vi "Main.vi"() -> ()   [LabVIEW 2017]
doc: "This template is for the Queued Message Handler design pattern.\n\nThe Event Handling Loop generates messages based on user interface actions.\n\nThe Message Handling Loop processes messages generated by the Event Handling Loop, or by other messages. The messages are string values, so new messages can be added easily to the Message Cases case structure in the Message Handling Loop. Each message cluster can also provide an optional value for Message Data, which is a variant that can be converted to whatever message-specific data is required."
uses:
  Position Slider.ctl
  Entry Display Data.ctl
  support/Message Queue/Enqueue Message (Single).vi
  <vilib>/Utility/error.llb/Error Cluster From Error Code.vi
  <vilib>/ErrorRing/Error Ring.xnode
  support/Message Queue/Message Queue.lvlib
  support/User Event - Stop/User Event - Stop.lvlib
panel:
  in  "Car Position Slider":T1 scale=0.0..4.0
  in  "Start":bool
  in  "Air Dry":bool
  in  "Tire Shine Foam":bool
  in  "Spot Free Rinse":bool
  in  "Low Pressure Wax":bool
  in  "High Pressure Wash":bool
  in  "Pre-Soak":bool
  in  "Bug Remover":bool
  in  "Under Body Wash":bool
  in  "Do Something Else <Replace Me>":bool
  in  "Do Something <Replace Me>":bool
  in  "Exit":bool
  # "These controls have associated \"Value Changed\" events configured in the Event Structure on the diagram.\n\nReplace them (and reconfigure the Event Structure) with the controls you need for your application."
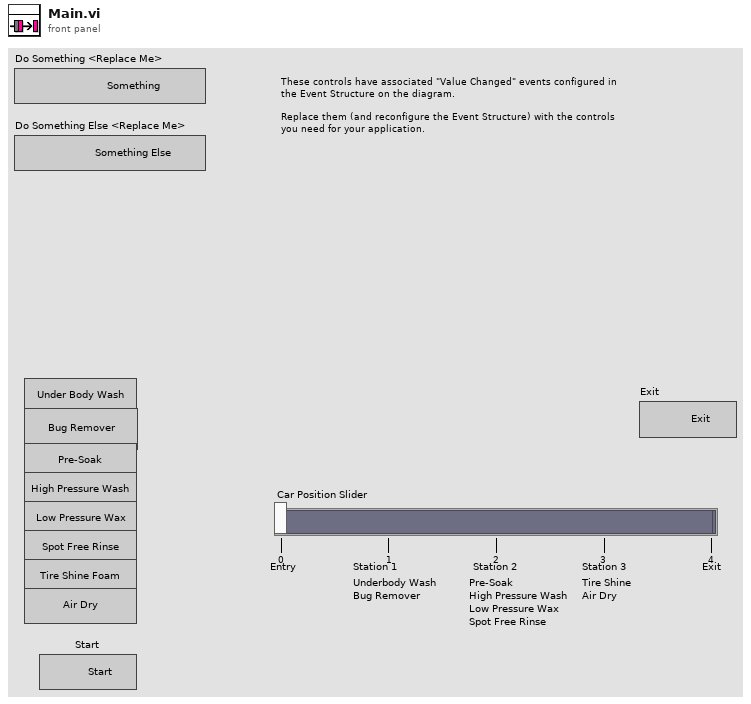
[diagram p1: front panel]
types:
  T1 = typedef "Position Slider.ctl" = i32
  T2 = typedef "Entry Display Data.ctl" = cluster{"Under Body Wash":bool, "Bug Remover":bool, "Pre-soak":bool, " High Pressure Wash":bool, "Low Pressure  Wax":bool, "Spot Free Rinse":bool, " Tire Shine Foam":bool, " Air Dry":bool, "Vehicle Postion":bool, "Wash Entry Display":bool, "Car Position Slider":T1}
  T3 = typedef "Message Queue.lvlib/All Message Queues.ctl" = cluster{"MHL":refnum<queue>, "Controller":refnum<queue>, "Display":refnum<queue>}
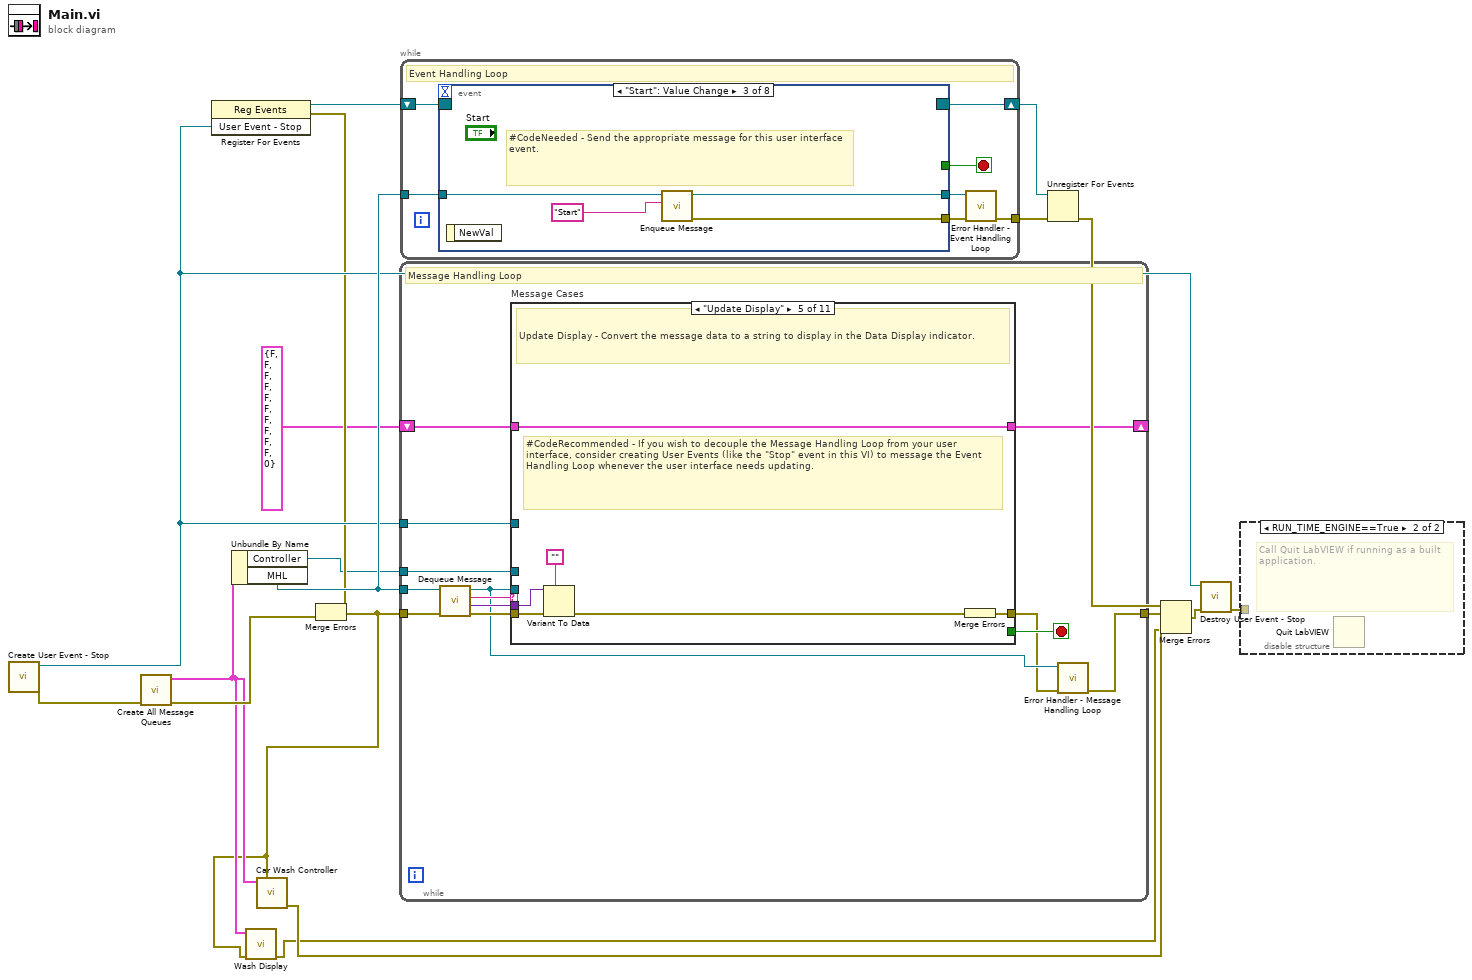
[diagram p0: block diagram]
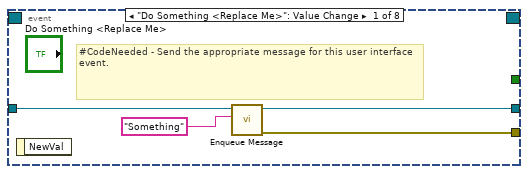
[diagram p3: hidden frame]
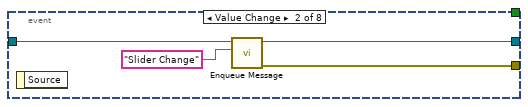
[diagram p4: hidden frame]
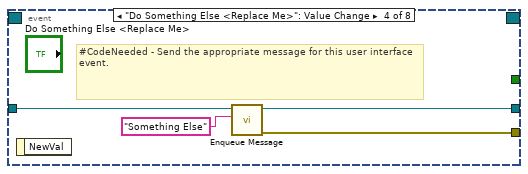
[diagram p5: hidden frame]
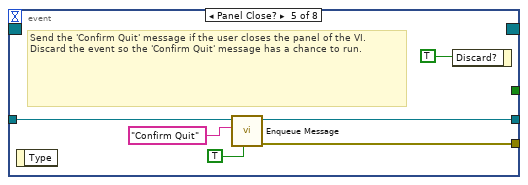
[diagram p6: hidden frame]
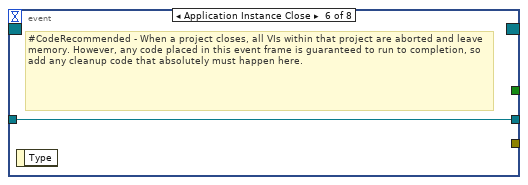
[diagram p7: hidden frame]
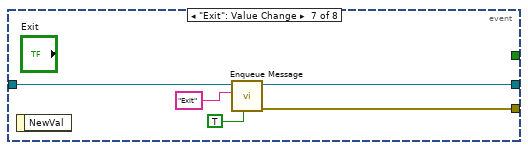
[diagram p8: hidden frame]
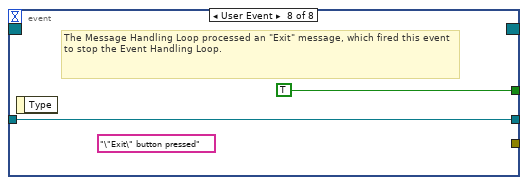
[diagram p9: hidden frame]
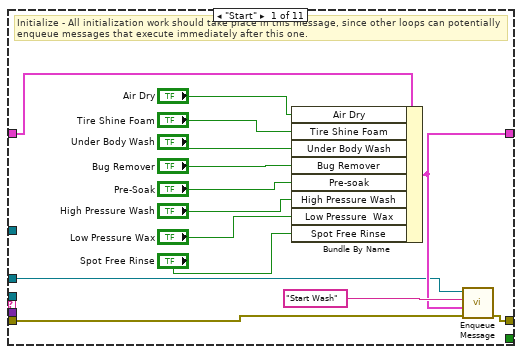
[diagram p10: hidden frame]
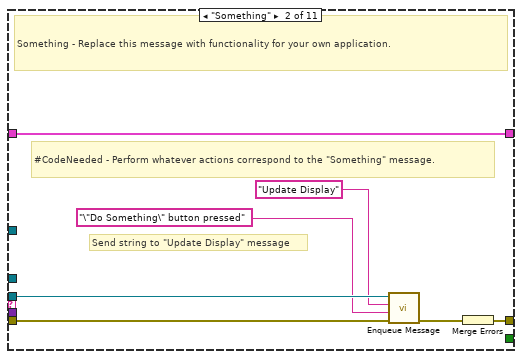
[diagram p11: hidden frame]
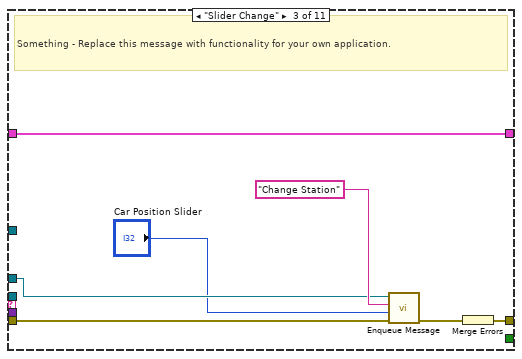
[diagram p12: hidden frame]
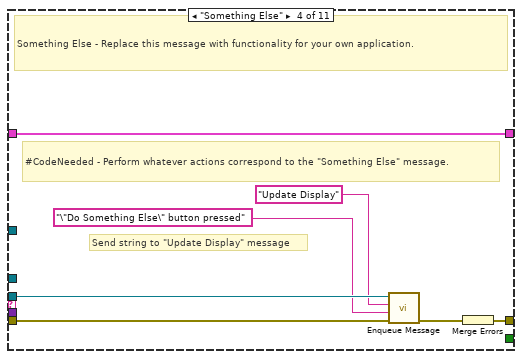
[diagram p13: hidden frame]
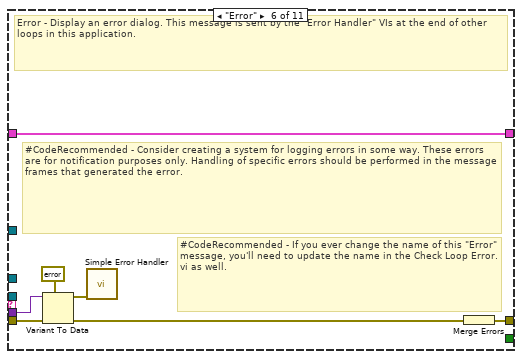
[diagram p14: hidden frame]
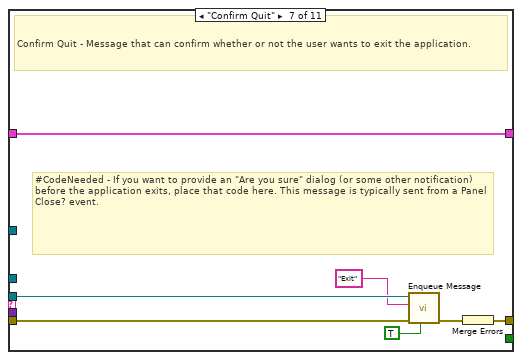
[diagram p15: hidden frame]
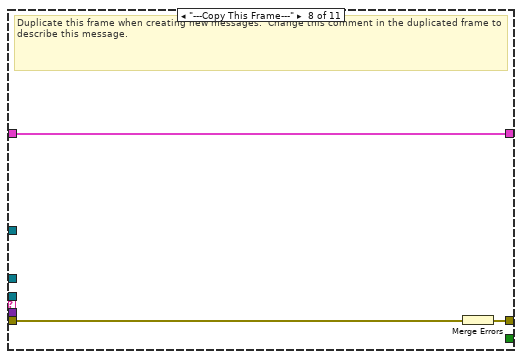
[diagram p16: hidden frame]
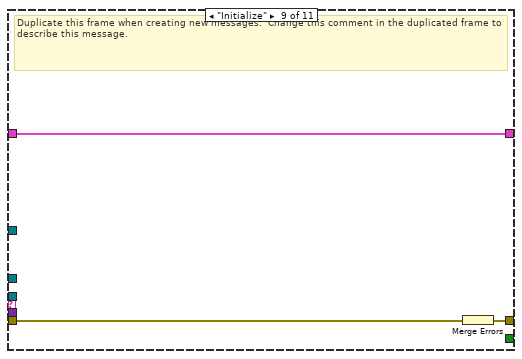
[diagram p17: hidden frame]
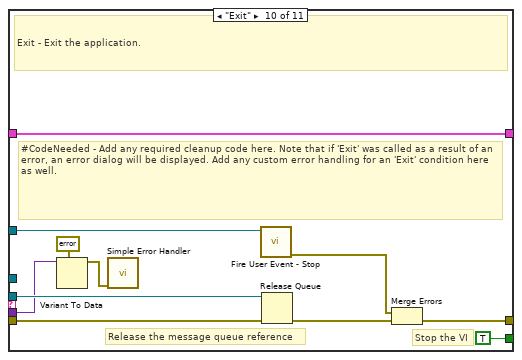
[diagram p18: hidden frame]
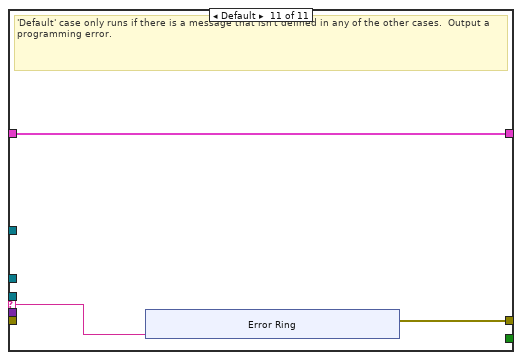
[diagram p19: hidden frame]
diagram:
  n1 = call "Create User Event - Stop.vi"() -> ("error out"=w16:errorcluster, "User Event - Stop"=w9:refnum<user-event>)  [unwired: 10 in]
  n2 = call "Create All Message Queues.vi"("error in (no error)"=w16) -> ("error out"=w6:errorcluster, "Message Queues out"=w4:T3)  [unwired: 9 in]
  n3 = register-events(w9) -> (reference out=w10:refnum<event-registration>, error out=w8:errorcluster)  [unwired: 2 in]
  n4 = Unbundle By Name(w4) -> ("Controller"=w7:refnum<queue>, "MHL"=w17:refnum<queue>)
  n5 = Merge Errors(w8, w6) -> (w2:errorcluster)
  n6 = call "Wash Display.vi"("error in (no error)"=w2, "Message Queues"=w4) -> ("error out"=w1:errorcluster)  [unwired: 9 in]
  n7 = call "Car Wash Controller.vi"("error in (no error)"=w2, "Message Queues"=w4) -> ("error out"=w5:errorcluster)  [unwired: 9 in]
  n8 = while {
    tunnel: w17 -> [w23]
    shift-right: [w30] -> _
    shift-left: T2 {"Under Body Wash"=FALSE, "Bug Remover"=FALSE, "Pre-soak"=FALSE, " High Pressure Wash"=FALSE, "Low Pressure  Wax"=FALSE, "Spot Free Rinse"=FALSE, " Tire Shine Foam"=FALSE, " Air Dry"=FALSE, "Vehicle Postion"=FALSE, "Wash Entry Display"=FALSE, "Car Position Slider"=0} ("Cluster") -> [w31]
    tunnel: w9 -> [w28]
    tunnel: w2 -> [w27]
    tunnel: [w21] -> w18
    tunnel: w7 -> [w19]
    stop <- w29 stop-if-true
    # "Message Handling Loop"
    n9 = call "Dequeue Message.vi"("error in (no error)"=w27, "Message Queue"=w23) -> ("error out"=w26:errorcluster, "Message Data"=w24:variant, "Message"=w25:string, "dup Message Queue"=w22:refnum<queue>)  [unwired: 6 in]
    n10 = case "Message Cases" shown="\"Update Display\"" w25 {
      selector: w25 -> [_ _ _ _ _ _ _ _ _ _ w104]
      tunnel: w22 -> [_ w48 _ w62 _ _ w82 _ _ w103 _]
      tunnel: w26 -> [w44 w50 w58 w64 w70 w79 w86 w89 w92 w96 _]
      tunnel: [w45 w51 w59 w65 w71 w73 w84 w87 w90 w99 w105] -> w20
      tunnel: w31 -> [w34 w52 w55 w66 w72 w78 w85 w88 w91 w102 w106]
      tunnel: [w33 w52 w55 w66 w72 w78 w85 w88 w91 w102 w106] -> w30
      tunnel: [_ _ _ _ _ _ _ _ _ TRUE _] -> w29
      tunnel: w24 -> [_ _ _ _ w69 w77 _ _ _ w93 _]
      tunnel: w28 -> [_ _ _ _ _ _ _ _ _ w98 _]
      tunnel: w19 -> [w32 _ w54 _ _ _ _ _ _ _ _]
      frame "Start" {
        # "Initialize - All initialization work should take place in this message, since other loops can potentially enqueue messages that execute immediately after this one."
        n11 = Bundle By Name(cluster=w34, "Air Dry"="Air Dry", "Tire Shine Foam"="Tire Shine Foam", "Under Body Wash"="Under Body Wash", "Bug Remover"="Bug Remover", "Pre-soak"="Pre-Soak", "High Pressure Wash"="High Pressure Wash", "Low Pressure  Wax"="Low Pressure Wax", "Spot Free Rinse"="Spot Free Rinse") -> (w33:T2)
        n12 = call-poly "Enqueue Message.vi"("error in (no error)"=w44, "Message Data"=w33, "Message"="Start Wash", "Message Queue"=w32) -> ("error out"=w45:errorcluster)  [unwired: 6 in, 1 out]
      }
      frame "Something" {
        # "Send string to \"Update Display\" message"
        # "#CodeNeeded - Perform whatever actions correspond to the \"Something\" message."
        # "Something - Replace this message with functionality for your own application."
        n13 = call-poly "Enqueue Message.vi"("error in (no error)"=w50, "Message Data"="\"Do Something\" button pressed" ("\"Do Something\" button pressed"), "Message"="Update Display", "Message Queue"=w48) -> ("error out"=w49:errorcluster)  [unwired: 6 in, 1 out]
        n14 = Merge Errors(w49) -> (w51:errorcluster)
      }
      frame "Slider Change" {
        # "Something - Replace this message with functionality for your own application."
        n15 = call-poly "Enqueue Message.vi"("error in (no error)"=w58, "Message Data"="Car Position Slider", "Message"="Change Station", "Message Queue"=w54) -> ("error out"=w57:errorcluster)  [unwired: 6 in, 1 out]
        n16 = Merge Errors(w57) -> (w59:errorcluster)
      }
      frame "Something Else" {
        # "Send string to \"Update Display\" message"
        # "#CodeNeeded - Perform whatever actions correspond to the \"Something Else\" message."
        # "Something Else - Replace this message with functionality for your own application."
        n17 = call-poly "Enqueue Message.vi"("error in (no error)"=w64, "Message Data"="\"Do Something Else\" button pressed" ("\"Do Something Else\" button pressed"), "Message"="Update Display", "Message Queue"=w62) -> ("error out"=w63:errorcluster)  [unwired: 6 in, 1 out]
        n18 = Merge Errors(w63) -> (w65:errorcluster)
      }
      frame "Update Display" {
        # "#CodeRecommended - If you wish to decouple the Message Handling Loop from your user interface, consider creating User Events (like the \"Stop\" event in this VI) to message the Event Handling Loop whenever the user interface needs updating."
        # "Update Display - Convert the message data to a string to display in the Data Display indicator."
        n19 = Variant To Data(error in=w70, type="", Variant=w69) -> (error out=w67:errorcluster)  [unwired: 1 out]
        n20 = Merge Errors(w67) -> (w71:errorcluster)
      }
      frame "Error" {
        # "#CodeRecommended - If you ever change the name of this \"Error\" message, you'll need to update the name in the Check Loop Error.vi as well."
        # "#CodeRecommended - Consider creating a system for logging errors in some way. These errors are for notification purposes only. Handling of specific errors should be performed in the message frames that generated the error."
        # "Error - Display an error dialog. This message is sent by the \"Error Handler\" VIs at the end of other loops in this application."
        n21 = Variant To Data(error in=w79, type=errorcluster {"status"=FALSE, "code"=0, "source"=""} ("error constant"), Variant=w77) -> (data=w75:errorcluster, error out=w74:errorcluster)
        n22 = call <vilib>:"Simple Error Handler.vi"("error in (no error)"=w75) -> ()  [unwired: 4 in, 5 out]
        n23 = Merge Errors(w74) -> (w73:errorcluster)
      }
      frame "Confirm Quit" {
        # "#CodeNeeded - If you want to provide an \"Are you sure\" dialog (or some other notification) before the application exits, place that code here. This message is typically sent from a Panel Close? event."
        # "Confirm Quit - Message that can confirm whether or not the user wants to exit the application."
        n24 = call-poly "Enqueue Message.vi"("Priority Message? (F)"=TRUE, "error in (no error)"=w86, "Message"="Exit", "Message Queue"=w82) -> ("error out"=w83:errorcluster)  [unwired: 6 in, 1 out]
        n25 = Merge Errors(w83) -> (w84:errorcluster)
      }
      frame "---Copy This Frame---" {
        # "Duplicate this frame when creating new messages.  Change this comment in the duplicated frame to describe this message."
        n26 = Merge Errors(w89) -> (w87:errorcluster)
      }
      frame "Initialize" {
        # "Duplicate this frame when creating new messages.  Change this comment in the duplicated frame to describe this message."
        n27 = Merge Errors(w92) -> (w90:errorcluster)
      }
      frame "Exit" {
        # "Stop the VI"
        # "Release the message queue reference"
        # "#CodeNeeded - Add any required cleanup code here. Note that if 'Exit' was called as a result of an error, an error dialog will be displayed. Add any custom error handling for an 'Exit' condition here as well."
        # "Exit - Exit the application."
        n28 = Variant To Data(type=errorcluster {"status"=FALSE, "code"=0, "source"=""} ("error constant"), Variant=w93) -> (data=w94:errorcluster)  [unwired: 1 in, 1 out]
        n29 = call <vilib>:"Simple Error Handler.vi"("error in (no error)"=w94) -> ()  [unwired: 4 in, 5 out]
        n30 = call "Fire User Event - Stop.vi"("User Event - Stop"=w98) -> ("error out"=w97:errorcluster)  [unwired: 10 in]
        n31 = Release Queue(queue=w103, error in (no error)=w96) -> (error out=w100:errorcluster)  [unwired: 1 in, 2 out]
        n32 = Merge Errors(w97, w100) -> (w99:errorcluster)
      }
      frame Default {
        # "'Default' case only runs if there is a message that isn't defined in any of the other cases.  Output a programming error."
        n33 = xnode "Error Ring"("parameter 0"=w104) -> ("error out"=w105:errorcluster)
      }
    }
    n34 = call "Error Handler - Message Handling Loop.vi"("error in (no error)"=w20, "Message Queue"=w22) -> ("dup error in"=w21:errorcluster)  [unwired: 8 in, 1 out]
  }
  n35 = while {
    tunnel: w17 -> [w120]
    shift-right: [w118] -> w13
    shift-left: w10 -> [w119]
    tunnel: [w114] -> w11
    stop <- w116 stop-if-true
    # "Event Handling Loop"
    n36 = event shown="[2] \"Start\": Value Change" {
      selector: w119 -> [_ _ _ _ _ _ _ _]
      dyn-events: [_ _ _ _ _ _ _ _] -> w118
      timeout: _ -> [_ _ _ _ _ _ _ _]
      tunnel: [_ _ _ _ _ _ _ TRUE ("Discard?")] -> w116
      tunnel: w120 -> [w124 w128 w132 w136 w141 w143 w148 w150]
      tunnel: [w121 w125 w129 w133 w140 _ w147 _] -> w117
      tunnel: [w123 w127 w131 w135 w139 w143 w146 w150] -> w115
      event "Do Something <Replace Me>": Value Change {
        # "#CodeNeeded - Send the appropriate message for this user interface event."
        n37 = event-data() -> ()  [unwired: 1 in, 1 out]
        n38 = call-poly "Enqueue Message.vi"("Message"="Something", "Message Queue"=w124) -> ("error out"=w121:errorcluster, "dup Message Queue"=w123:refnum<queue>)  [unwired: 8 in]
      }
      event Value Change {
        n39 = event-data() -> ()  [unwired: 1 in, 1 out]
        n40 = call-poly "Enqueue Message.vi"("Message"="Slider Change", "Message Queue"=w128) -> ("error out"=w125:errorcluster, "dup Message Queue"=w127:refnum<queue>)  [unwired: 8 in]
      }
      event "Start": Value Change {
        # "#CodeNeeded - Send the appropriate message for this user interface event."
        n41 = event-data() -> ()  [unwired: 1 in, 1 out]
        n42 = call-poly "Enqueue Message.vi"("Message"="Start", "Message Queue"=w132) -> ("error out"=w129:errorcluster, "dup Message Queue"=w131:refnum<queue>)  [unwired: 8 in]
      }
      event "Do Something Else <Replace Me>": Value Change {
        # "#CodeNeeded - Send the appropriate message for this user interface event."
        n43 = event-data() -> ()  [unwired: 1 in, 1 out]
        n44 = call-poly "Enqueue Message.vi"("Message"="Something Else", "Message Queue"=w136) -> ("error out"=w133:errorcluster, "dup Message Queue"=w135:refnum<queue>)  [unwired: 8 in]
      }
      event Panel Close? {
        # "Send the 'Confirm Quit' message if the user closes the panel of the VI. Discard the event so the 'Confirm Quit' message has a chance to run."
        n45 = event-data() -> ()  [unwired: 1 in, 1 out]
        n46 = call-poly "Enqueue Message.vi"("Priority Message? (F)"=TRUE, "Message"="Confirm Quit", "Message Queue"=w141) -> ("error out"=w140:errorcluster, "dup Message Queue"=w139:refnum<queue>)  [unwired: 7 in]
        n47 = event-data("Discard?"=TRUE) -> ()  [unwired: 1 in, 1 out]
      }
      event Application Instance Close {
        # "#CodeRecommended - When a project closes, all VIs within that project are aborted and leave memory. However, any code placed in this event frame is guaranteed to run to completion, so add any cleanup code that absolutely must happen here."
        n48 = event-data() -> ()  [unwired: 1 in, 1 out]
      }
      event "Exit": Value Change {
        n49 = event-data() -> ()  [unwired: 1 in, 1 out]
        n50 = call-poly "Enqueue Message.vi"("Priority Message? (F)"=TRUE, "Message"="Exit", "Message Queue"=w148) -> ("error out"=w147:errorcluster, "dup Message Queue"=w146:refnum<queue>)  [unwired: 7 in]
      }
      event User Event {
        (unwired) "\"Exit\" button pressed" ("VI Stopped")
        # "The Message Handling Loop processed an \"Exit\" message, which fired this event to stop the Event Handling Loop."
        n51 = event-data() -> ()  [unwired: 1 in, 1 out]
      }
    }
    n52 = call "Error Handler - Event Handling Loop.vi"("error in (no error)"=w117, "Message Queue"=w115) -> ("dup error in"=w114:errorcluster)  [unwired: 8 in, 1 out]
  }
  n53 = Unregister For Events(event registration refnum=w13, error in=w11) -> (error out=w14:errorcluster)
  n54 = Merge Errors(w14, w18, w5, w1) -> (w15:errorcluster)
  n55 = call "Destroy User Event - Stop.vi"("error in (no error)"=w15, "User Event - Stop"=w9) -> ("error out"=w12:errorcluster)  [unwired: 9 in]
  n56 = disable-structure shown="RUN_TIME_ENGINE==True" {
    disable-tunnel: w12 -> [_ _]
    frame condition #0 (active) {
    }
    frame condition #1 {
      # "Call Quit LabVIEW if running as a built application."
      n57 = Quit LabVIEW() -> ()  [unwired: 1 in]
    }
  }
